vi "Obtain.vi"(5 "Timeout (10000 ms)":i32=10000, 7 "port (15000)":u16=15000, 8 "Error In":errorcluster, 9 "Cmd Line Mode (Hidden)":T1=enum."Hidden", 10 "Python Executable (empty)":path, 11 ".py File":path) -> (0 "Error Out":errorcluster, 3 "OPI Ref":refnum<data-value>)   [LabVIEW 2019, in "OPI.lvclass"]
doc: "Obtain reference to Open Python Interface. The reference represents the local address to Python Execution Server, the local memory used to store arguments, return values and exception info from function calls. \n\nThe .py File input allows you to execute preexisting .py code to set variable values, define functions etc.\n\nEach Obtain method launches a seperate thread on PES (Python Execution Server). This means all values and methods will be local to it. You can create as many seperate OPI references as needed, but they will only be able to communicate through LabVIEW.\n\nSpliting the OPI reference wire is supported and will be handled correctly, allowing access to the same PES Client Handler thread. Each parallel call will however block and wait until previous call returns.\n\nYou can specify the path to your python executable if it's not registered with the operating system, or if you want to use other version."
uses:
  OPI.lvclass
  Typedefs/Cmd Line Mode.ctl
  OPI.lvclass/OPI.ctl
  <vilib>/Utility/error.llb/Error Cluster From Error Code.vi
  <vilib>/ErrorRing/Error Ring.xnode
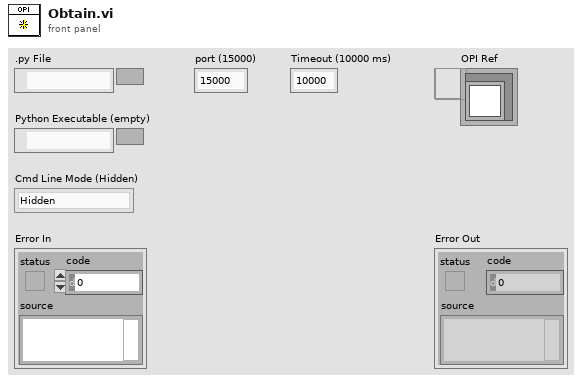
[diagram p1: front panel]
types:
  T1 = typedef "OPI.lvclass/Cmd Line Mode.ctl" = enum16{"Debug", "Hidden"}
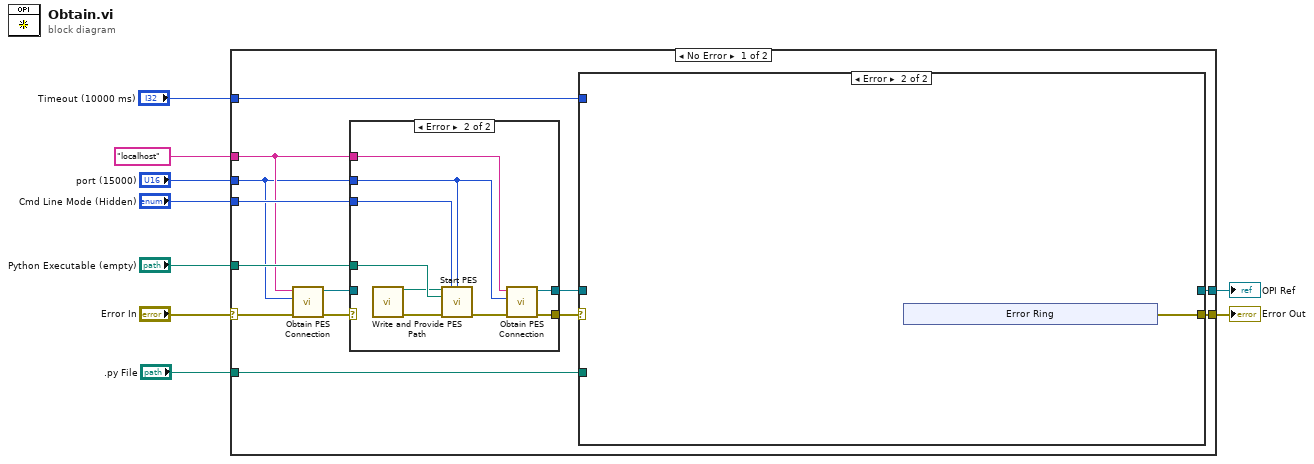
[diagram p0: block diagram]
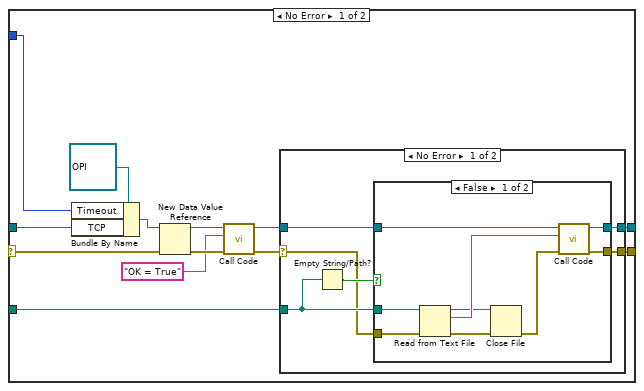
[diagram p2: hidden frame]
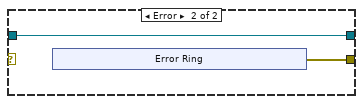
[diagram p4: hidden frame]
diagram:
  n1 = case shown="No Error" "Error In" {
    selector: "Error In" -> [w10 w77]
    tunnel: "Cmd Line Mode (Hidden)" -> [w22 _]
    tunnel: "Python Executable (empty)" -> [w21 _]
    tunnel: "localhost" ("address") -> [w18 _]
    tunnel: "port (15000)" -> [w17 _]
    tunnel: [w15 _] -> w5
    tunnel: [w14 w77] -> w4
    tunnel: "Timeout (10000 ms)" -> [w13 _]
    tunnel: ".py File" -> [w12 _]
    frame No Error {
      n2 = call "Obtain PES Connection.vi"("Error In"=w10, "port"=w17, "address"=w18) -> ("Error Out"=w20:errorcluster, "TCP Out"=w19:refnum<k5>)  [unwired: 7 in]
      n3 = case shown="Error" w20 {
        selector: w20 -> [w66 _]
        tunnel: [w66 w70] -> w11
        tunnel: w22 -> [_ w76]
        tunnel: w21 -> [_ w75]
        tunnel: w17 -> [_ w72]
        tunnel: [w67 w71] -> w16
        tunnel: w19 -> [w67 _]
        tunnel: w18 -> [_ w73]
        frame No Error {
        }
        frame Error {
          n4 = call "Write and Provide PES Path.vi"() -> ("Error Out"=w69:errorcluster, "PES File Path"=w68:path)  [unwired: 10 in]
          n5 = call "Start PES.vi"("Server .py Path"=w68, "Cmd Line Mode"=w76, "port"=w72, "Python Executable"=w75, "Error In"=w69) -> ("Error Out"=w74:errorcluster)  [unwired: 10 in]
          n6 = call "Obtain PES Connection.vi"("Error In"=w74, "port"=w72, "address"=w73) -> ("Error Out"=w70:errorcluster, "TCP Out"=w71:refnum<k5>)  [unwired: 7 in]
        }
      }
      n7 = case shown="Error" w11 {
        selector: w11 -> [w29 _]
        tunnel: w16 -> [w33 _]
        tunnel: [w32 _] -> w15
        tunnel: [w31 w60] -> w14
        tunnel: w13 -> [w28 _]
        tunnel: w12 -> [w30 _]
        frame No Error {
          n8 = Bundle By Name(cluster=refnum<class "OPI.lvclass"> refnum ("OPI in"), "Timeout"=w28, "TCP"=w33) -> (w34:refnum<class "OPI.lvclass">)
          n9 = New Data Value Reference(data value=w34, error in=w29) -> (data value reference=w27:refnum<data-value>, error out=w26:errorcluster)
          n10 = call "Call Code.vi"("Error In"=w26, "Pythonic Code"="OK = True", "OPI Ref"=w27) -> ("Error Out"=w23:errorcluster, "OPI Ref"=w25:refnum<data-value>)  [unwired: 7 in]
          n11 = case shown="No Error" w23 {
            selector: w23 -> [w36 _]
            tunnel: [w41 w53] -> w32
            tunnel: [w40 w54] -> w31
            tunnel: w30 -> [w39 _]
            tunnel: w25 -> [w37 w53]
            frame No Error {
              n12 = Empty String/Path?(string/path=w39) -> (empty?=w38:bool)
              n13 = case shown="False" w38 {
                tunnel: w37 -> [w50 w52]
                tunnel: w36 -> [w49 w51]
                tunnel: [w48 w52] -> w41
                tunnel: [w47 w51] -> w40
                tunnel: w39 -> [w45 _]
                frame False {
                  n14 = Read from Text File(file (use dialog)=w45, error in=w49) -> (refnum out=w44:refnum<file>, text=w46:string, error out=w43:errorcluster)  [unwired: 2 in, 1 out]
                  n15 = Close File(refnum=w44, error in=w43) -> (error out=w42:errorcluster)  [unwired: 1 out]
                  n16 = call "Call Code.vi"("Error In"=w42, "Pythonic Code"=w46, "OPI Ref"=w50) -> ("Error Out"=w47:errorcluster, "OPI Ref"=w48:refnum<data-value>)  [unwired: 7 in]
                }
                frame True {
                }
              }
            }
            frame Error {
              n17 = xnode "Error Ring"() -> ("error out"=w54:errorcluster)
            }
          }
        }
        frame Error {
          n18 = xnode "Error Ring"() -> ("error out"=w60:errorcluster)
        }
      }
    }
    frame Error {
    }
  }
  "Error Out" <- w4
  "OPI Ref" <- w5
